vi "Get Result.vi"(8 "error in (no error)":errorcluster, 11 "LR-700 in":refnum<class "LR-700 Driver.lvclass">=refnum) -> (0 "error out":errorcluster, 2 "Result":refnum<class "Acquired Result.lvclass">, 3 "LR-700 out":refnum<class "LR-700 Driver.lvclass">)   [LabVIEW 2016, in "LR-700 Driver.lvclass"]
uses:
  LR-700 Driver.lvclass
  C:/github/NHMFL_Core/Libraries/Instruments/VISA Instrument/VISA Instrument.lvclass
  C:/github/NHMFL_Core/Libraries/Instruments/Instrument Driver/Channel Scanner Driver/Channel Scanner Driver.lvclass
  C:/github/NHMFL_Core/Libraries/Instruments/Instrument Driver/Instrument Driver.lvclass
  Results/Acquired Result/Acquired Result.lvclass
  Results/Acquired Result/Acquired Result.lvclass/Acquired Result.ctl
  VISA Instrument/VISA Instrument.lvclass/VISA Instrument.ctl
  Instrument Driver/Channel Scanner Driver/Channel Scanner Driver.lvclass/Channel Scanner Driver.ctl
  Instrument Driver/Instrument Driver.lvclass/Instrument Driver.ctl
  Results/Acquired Result/Read Group.vi
  VISA Instrument/Read VISA resource.vi
  Instrument Driver/Channel Scanner Driver/Read Scan Channels.vi
  Instrument Driver/Read Recorder name.vi
  Instrument Driver/Read Cycle count.vi
  Instrument Driver/Channel Scanner Driver/Read Next channel idx.vi
  Instrument Driver/Read Cycle period.vi
  VISA Instrument/Write VISA resource.vi
  Results/Acquired Result/Write Group.vi
  Results/Acquired Result/Write Time group.vi
  Results/Acquired Result/Write Time value.vi
  <vilib>/express/express shared/transition.llb/Dynamic To Waveform Array.vi
  <vilib>/express/express signal manip/GetorSetDDTAttributes/Set DDT Attributes/SetT0.vi
  <vilib>/express/express shared/transition.llb/Waveform Array To Dynamic.vi
  <vilib>/express/express signal manip/GetorSetDDTAttributes/Set DDT Attributes/Set DDT Properties.xnode
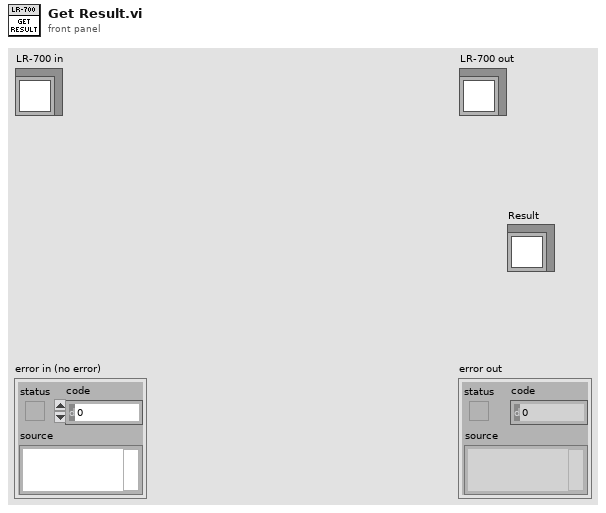
[diagram p1: front panel]
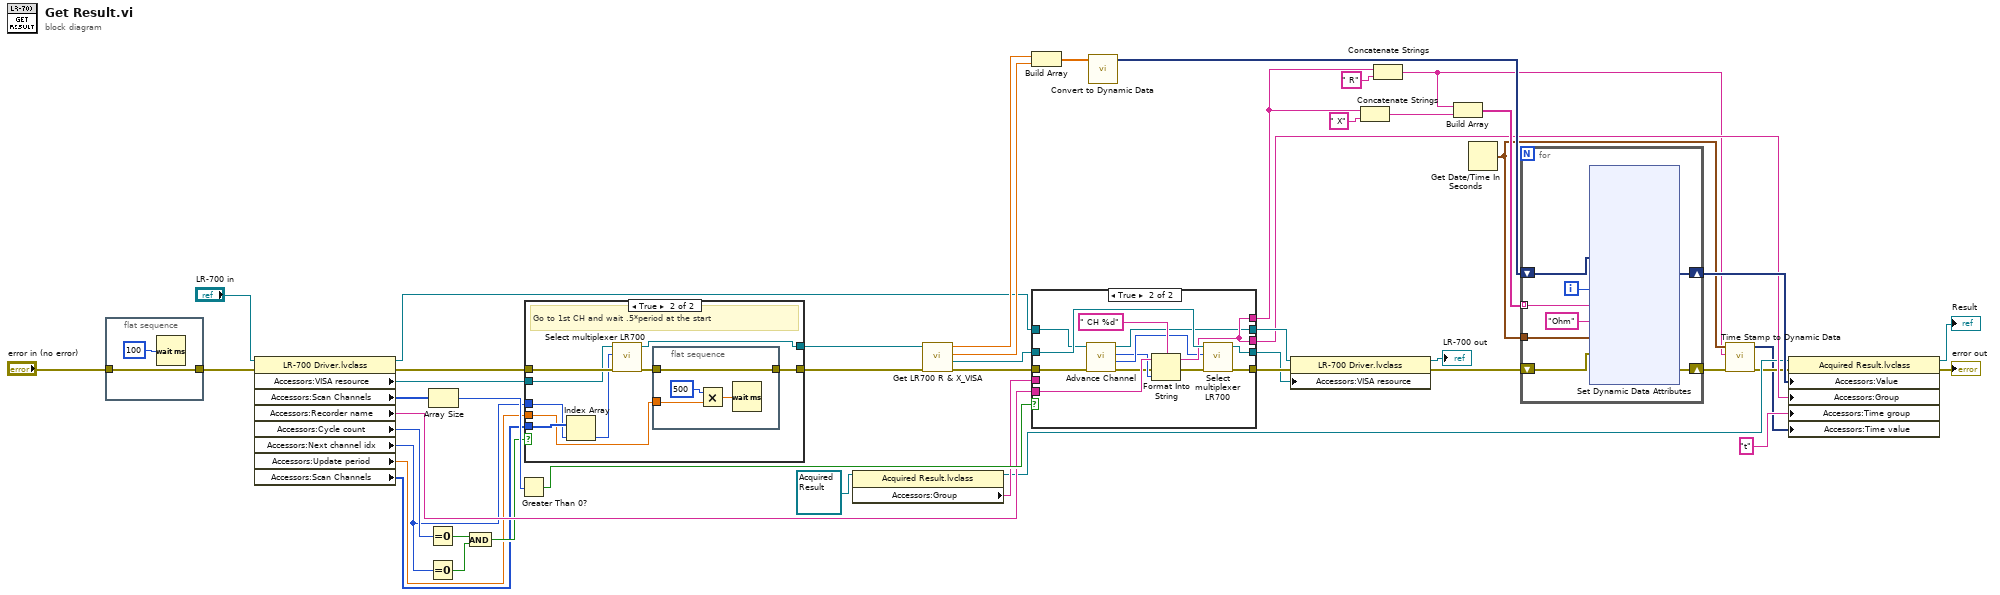
[diagram p0: block diagram]
diagram:
  n1 = flat-sequence {
    tunnel: "error in (no error)" -> [w50]
    tunnel: [w50] -> w38
    frame #0 {
      n2 = Wait (ms)(milliseconds to wait=u32 100) -> ()  [unwired: 1 out]
    }
  }
  n3 = property class="LR-700 Driver.lvclass"(reference="LR-700 in", error in=w38) -> (reference out=w37:refnum<class "LR-700 Driver.lvclass">, error out=w7:errorcluster, "Accessors:VISA resource"=w4:refnum<visa-resource-name>, "Accessors:Scan Channels"=w34:i32[], "Accessors:Recorder name"=w33:string, "Accessors:Cycle count"=w10:i32, "Accessors:Next channel idx"=w5:i32, "Accessors:Update period"=w1:dbl, "Accessors:Scan Channels"=w6:i32[])
  n4 = Equal To 0?(x=w10) -> (x = 0?=w11:bool)
  n5 = Equal To 0?(x=w5) -> (x = 0?=w8:bool)
  n6 = Array Size(array=w34) -> (size(s)=w44:i32)
  n7 = And(x=w11, y=w8) -> (x .and. y?=w9:bool)
  n8 = Greater Than 0?(x=w44) -> (x > 0?=w41:bool)
  n9 = case shown="True" w9 {
    tunnel: w7 -> [w51 w61]
    tunnel: w6 -> [_ w60]
    tunnel: w5 -> [_ w59]
    tunnel: w4 -> [w52 w58]
    tunnel: [w52 w57] -> w3
    tunnel: [w51 w55] -> w2
    tunnel: w1 -> [_ w53]
    frame False {
      # "Do nothing"
    }
    frame True {
      # "Go to 1st CH and wait .5*period at the start"
      n10 = Index Array(array=w60, index=w59) -> (element=w54:i32)
      n11 = call "Select multiplexer LR700.vi"("error in"=w61, "Sensor"=w54, "VISA Resource Name"=w58) -> ("error out"=w56:errorcluster, "VISA Resource Name Out"=w57:refnum<visa-resource-name>)  [unwired: 7 in]
      n12 = flat-sequence {
        tunnel: w56 -> [w65]
        tunnel: [w65] -> w55
        tunnel: w53 -> [w62]
        frame #0 {
          n13 = Multiply(x=u32 500 ("milliseconds to wait"), y=w62) -> (x*y=w63:dbl)
          n14 = Wait (ms)(milliseconds to wait=w63) -> ()  [unwired: 1 out]
        }
      }
    }
  }
  n15 = property class="Acquired Result.lvclass"(reference=refnum<class "Acquired Result.lvclass"> refnum ("Result")) -> (reference out=w18:refnum<class "Acquired Result.lvclass">, "Accessors:Group"=w19:string)  [unwired: 1 in, 1 out]
  n16 = call "Get LR700 R & X_VISA.vi"("error in (no error)"=w2, "VISA resource name"=w3) -> ("error out"=w43:errorcluster, "VISA resource name out"=w47:refnum<visa-resource-name>, "X"=w45:dbl, "Resistance"=w46:dbl)  [unwired: 2 in]
  n17 = Build Array(w46, w45) -> (w32:dbl[])
  n18 = case shown="True" w41 {
    tunnel: w47 -> [w70 w79]
    tunnel: [w70 w78] -> w35
    tunnel: w37 -> [w67 w76]
    tunnel: w33 -> [w69 w83]
    tunnel: [w69 w77] -> w22
    tunnel: w43 -> [w68 w72]
    tunnel: [w68 w80] -> w42
    tunnel: [w67 w75] -> w36
    tunnel: [w66 w77] -> w21
    tunnel: w19 -> [w66 _]
    frame False {
    }
    frame True {
      n19 = call-dynamic "Advance Channel.vi"("error in (no error)"=w72, "Channel Scanner Driver in"=w76) -> ("error out"=w71:errorcluster, "Next channel"=w74:i32, "Current channel"=w73:i32, "Channel Scanner Driver out"=w75:refnum<class "LR-700 Driver.lvclass">)  [unwired: 6 in]
      n20 = Format Into String(format string=" CH %d", initial string=w83, error in=w71, w73) -> (resulting string=w77:string, error out=w81:errorcluster)
      n21 = call "Select multiplexer LR700.vi"("error in"=w81, "Sensor"=w74, "VISA Resource Name"=w79) -> ("error out"=w80:errorcluster, "VISA Resource Name Out"=w78:refnum<visa-resource-name>)  [unwired: 7 in]
    }
  }
  n22 = call "Convert to Dynamic Data"("Array"=w32) -> ("Dynamic Data Type"=w28:dynamicdata)  [unwired: 3 in]
  n23 = property class="LR-700 Driver.lvclass"(reference=w36, error in=w42, "Accessors:VISA resource"=w35) -> (reference out=→"LR-700 out":refnum<class "LR-700 Driver.lvclass">, error out=w26:errorcluster)
  n24 = Concatenate Strings(w22, " X") -> (w29:string)
  n25 = Concatenate Strings(w22, " R") -> (w12:string)
  n26 = Build Array(w12, w29) -> (w27:string[])
  n27 = Get Date/Time In Seconds() -> (seconds since 1Jan1904=w16:timestamp)
  n28 = for {
    shift-right: [w84] -> w23
    shift-left: w28 -> [w91]
    tunnel: w27 -> [w89] mode=indexing
    shift-right: [w85] -> w15
    shift-left: w26 -> [w86]
    tunnel: w16 -> [w87]
    i -> [w90]
    n29 = xnode "Set Dynamic Data Attributes"("Signals In"=w91, "Signal Index"=w90, "Signal Name"=w89, "Unit"="Ohm", "Timestamp"=w87, "error in"=w86) -> ("Signals Out"=w84:dynamicdata, "error out"=w85:errorcluster)
  }
  n30 = call "Time Stamp to Dynamic Data.vi"("Error In"=w15, "Name"=w12, "Time Stamp Control"=w16) -> ("Error Out"=w14:errorcluster, "Dynamic Data Type"=w13:dynamicdata)  [unwired: 7 in]
  n31 = property class="Acquired Result.lvclass"(reference=w18, error in=w14, "Accessors:Value"=w23, "Accessors:Group"=w21, "Accessors:Time group"="t" ("Time group"), "Accessors:Time value"=w13) -> (reference out=→"Result":refnum<class "Acquired Result.lvclass">, error out=→"error out":errorcluster)
